vi "Read Acq Interval.vi"(8 "error in (no error)":errorcluster, 11 "TRIG Next Acq Request in":refnum<class "TRIG Next Acq Request.lvclass">) -> (0 "error out":errorcluster, 2 "Acq Interval":dbl caption="Acq Interval, s", 3 "TRIG Next Acq Request out":refnum<class "TRIG Next Acq Request.lvclass">)   [LabVIEW 2019, in "Trig Process.lvlib" / "TRIG Next Acq Request.lvclass"]
uses:
  TRIG Next Acq Request.lvclass
  TRIG Next Acq Request.lvclass/TRIG Next Acq Request.ctl
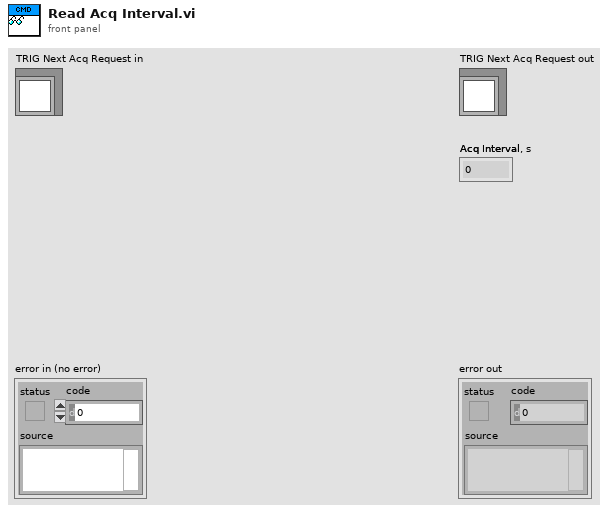
[diagram p1: front panel]
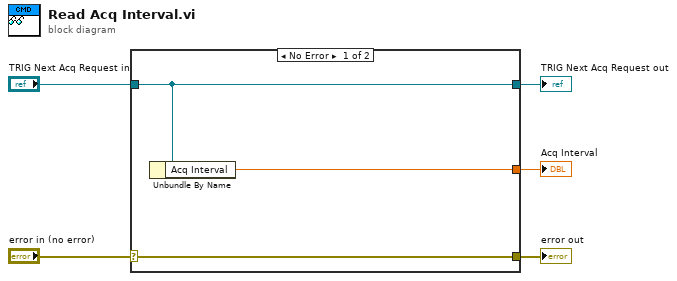
[diagram p0: block diagram]
diagram:
  n1 = case shown="No Error" "error in (no error)" {
    selector: "error in (no error)" -> [w8 w9]
    tunnel: [w8 w9] -> w4
    tunnel: [w7 w10] -> w2
    tunnel: "TRIG Next Acq Request in" -> [w7 w10]
    tunnel: [w6 _] -> w1
    frame No Error {
      n2 = Unbundle By Name(w7) -> ("Acq Interval"=w6:dbl)
    }
    frame Error {
    }
  }
  "error out" <- w4
  "TRIG Next Acq Request out" <- w2
  "Acq Interval" <- w1
